vi "Get Position.vi"(8 "error in (no error)":errorcluster, 11 "KUKA youBot arm motor_EtherCAT in":refnum<class "NI_Robotics_KUKA youBot Arm Motor_EtherCAT.lvclass">) -> (0 "error out":errorcluster, 2 "CCW position (rad)":dbl, 3 "KUKA youBot arm motor_EtherCAT out":refnum<class "NI_Robotics_KUKA youBot Arm Motor_EtherCAT.lvclass">)   [LabVIEW 2017, in "NI_Robotics_KUKA youBot Host.lvlib" / "NI_Robotics_KUKA youBot Arm Motor_EtherCAT.lvclass"]
uses:
  <vilib>/robotics/KUKA youBot/Motor/Arm Motor EtherCAT/NI_Robotics_KUKA youBot Arm Motor_EtherCAT.lvclass
  <vilib>/robotics/KUKA youBot/Motor/Arm Motor EtherCAT/NI_Robotics_KUKA youBot Arm Motor_EtherCAT.lvclass/NI_Robotics_KUKA youBot Arm Motor_EtherCAT.ctl
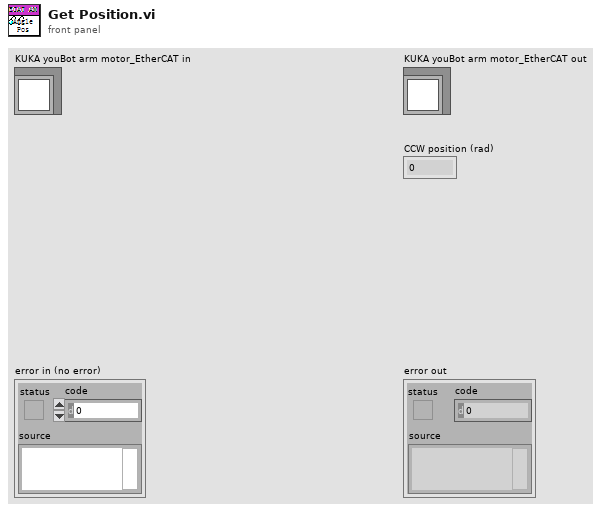
[diagram p1: front panel]
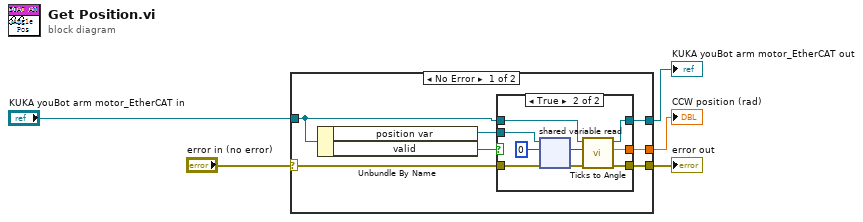
[diagram p0: block diagram]
diagram:
  n1 = case shown="No Error" "error in (no error)" {
    selector: "error in (no error)" -> [w11 w24]
    tunnel: "KUKA youBot arm motor_EtherCAT in" -> [w7 w25]
    tunnel: [w10 _] -> w3
    tunnel: [w6 w25] -> w2
    tunnel: [w9 w24] -> w1
    frame No Error {
      n2 = Unbundle By Name(w7) -> ("position var"=w12:refnum<k21>, "valid"=w8:bool)
      n3 = case shown="True" w8 {
        tunnel: w12 -> [_ w22]
        tunnel: w11 -> [w14 w21]
        tunnel: [_ w17] -> w10
        tunnel: [w14 w18] -> w9
        tunnel: w7 -> [w13 w16]
        tunnel: [w13 w15] -> w6
        frame False {
        }
        frame True {
          n4 = shared-variable-read(w22, w21, 0 ("data type")) -> (w19:errorcluster, w20:i32)  [unwired: 2 out]
          n5 = call <vilib>:"Ticks to Angle.vi"("error in (no error)"=w19, "ticks"=w20, "KUKA youBot arm motor_EtherCAT in"=w16) -> ("error out"=w18:errorcluster, "angle (radian)"=w17:dbl, "KUKA youBot arm motor_EtherCAT out"=w15:refnum<class "NI_Robotics_KUKA youBot Arm Motor_EtherCAT.lvclass">)  [unwired: 6 in]
        }
      }
    }
    frame Error {
    }
  }
  "error out" <- w1
  "KUKA youBot arm motor_EtherCAT out" <- w2
  "CCW position (rad)" <- w3
